vi "String to U8.vi"(8 "error in":errorcluster, 11 "Integer String":string) -> (0 "error out":errorcluster, 3 "U8":u8)   [LabVIEW 2020, in "CANopen.lvlib"]
doc: "A string that contains the number to convert."
uses:
  CANopen.lvlib
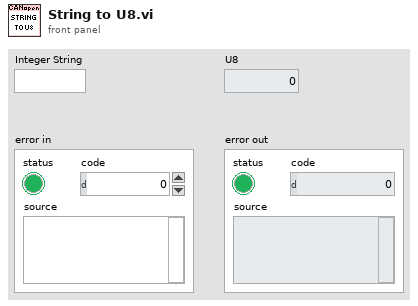
[diagram p1: front panel]
types:
  T1 = enum16{"U8", "U16", "U32", "I8", "I16", "I32", "I64", "U64"}
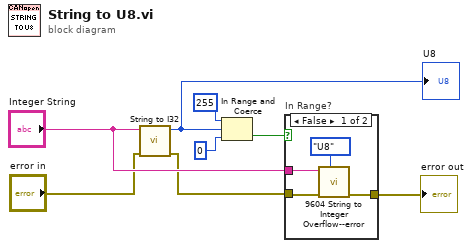
[diagram p0: block diagram]
diagram:
  n1 = call "String to I32.vi"("error in"="error in", "Integer String"="Integer String") -> ("error out"=w1:errorcluster, "I32"=w5:i32)  [unwired: 8 in]
  "U8" <- w5
  n2 = In Range and Coerce(upper limit=255, x=w5, lower limit=0) -> (In Range?=w6:bool)  [unwired: 1 out]
  n3 = case "In Range?" shown="False" w6 {
    tunnel: w1 -> [w12 w13]
    tunnel: [w11 w13] -> w4
    tunnel: "Integer String" -> [w10 _]
    frame False {
      n4 = call "9604 String to Integer Overflow--error.vi"("Type"=T1."U8", "error in"=w12, "Integer String"=w10) -> ("error out"=w11:errorcluster)  [unwired: 8 in]
    }
    frame True {
    }
  }
  "error out" <- w4
